vi "videotest.vi"   [LabVIEW 2014]
types:
  T1 = typedef "IMAQ Image.ctl" = refnum<image>
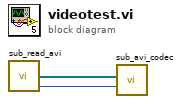
[diagram p0: block diagram]
diagram:
  n1 = call "sub_read_avi.vi"() -> ("Frames Per Second"=w1:u32, "image array"=w2:T1[])  [unwired: 4 in]
  n2 = call "sub_avi_codec.vi"("Frames Per Second"=w1, "image array"=w2) -> ()  [unwired: 10 in]
